vi "ev Scintilla KeyDown.vi"(4 "LF2R IDE in":refnum<class "LF2R IDE.lvclass">, 5 "Event Data":cluster{"sender":refnum<k24>, "e":refnum<k24>}, 6 "Control Ref":refnum<k24>, 7 "Event Common Data":T1) -> ()   [LabVIEW 2018, in "LF2R IDE.lvlib" / "LF2R IDE.lvclass"]
uses:
  LF2R IDE.lvclass
  D:/project/hobby/LabVIEW/LF2R/LabVIEW/Source/ScintillaNET/dll/ScintillaNET.dll
  ScintillaNET/dll/ScintillaNET.dll
  System.Windows.Forms
  C:/Program Files (x86)/National Instruments/LabVIEW 2018/vi.lib/ActorFramework/Actor/Actor.lvclass
  LF2R IDE Cmd.ctl
  <vilib>/ActorFramework/Actor/Actor.lvclass/Actor.ctl
  <vilib>/ActorFramework/Message Enqueuer/Message Enqueuer.lvclass/Message Enqueuer.ctl
  LF2R IDE Messages/LF2R IDE Cmd Msg/LF2R IDE Cmd Msg.lvclass/LF2R IDE Cmd Msg.ctl
  <vilib>/ActorFramework/Message Enqueuer/Init from Existing Queue.vi
  <vilib>/ActorFramework/Message Enqueuer/Enqueue.vi
  LF2R IDE Messages/LF2R IDE Cmd Msg/LF2R IDE Cmd Msg.lvclass
  C:/Program Files (x86)/National Instruments/LabVIEW 2018/vi.lib/ActorFramework/Message/Message.lvclass
  <vilib>/ActorFramework/Message Priority Queue/Priority Enqueue.vi
  <vilib>/ActorFramework/Message Enqueuer/Message Enqueuer.lvclass
  <vilib>/ActorFramework/Actor/Actor.lvclass
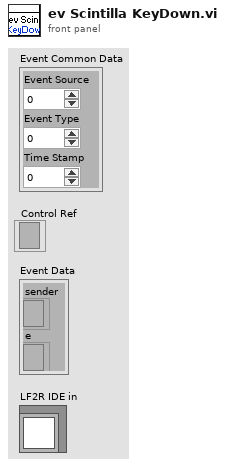
[diagram p1: front panel]
types:
  T1 = cluster{"Event Source":i32, "Event Type":u32, "Time Stamp":u32}
  T2 = typedef "LF2R IDE.lvlib/LF2R IDE.lvclass/LF2R IDE Cmd.ctl" = enum16{"Save Data File", "Write Configuration", "Save Configuration", "Update Frame Image"}
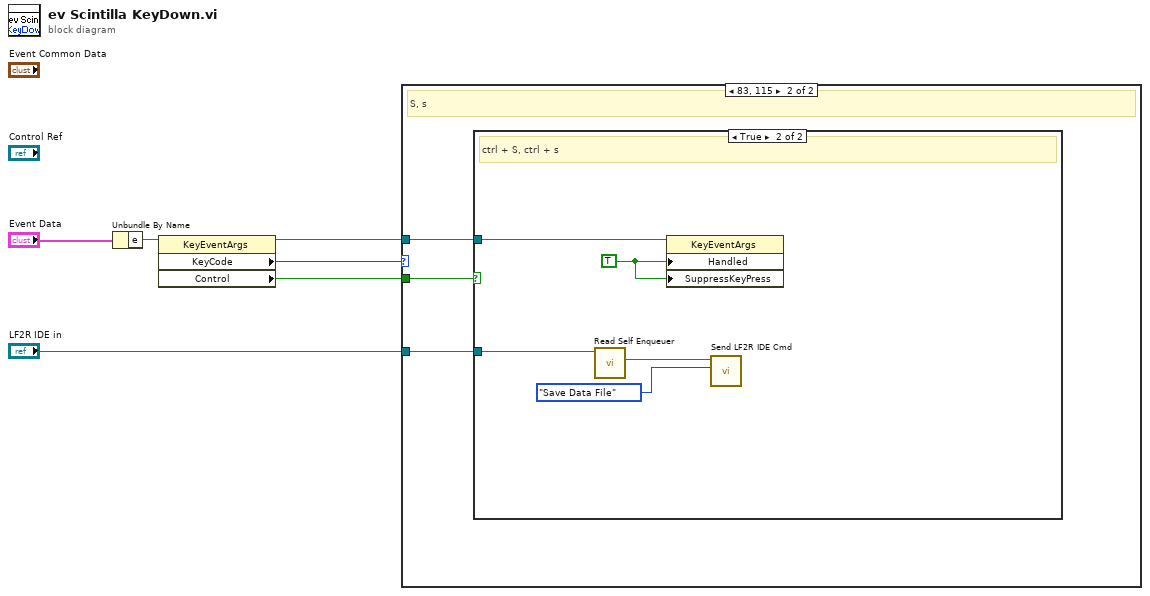
[diagram p0: block diagram]
diagram:
  n1 = Unbundle By Name("Event Data") -> ("e"=w6:refnum<k24>)
  n2 = property class="KeyEventArgs"(reference=w6) -> (reference out=w3:refnum<k24>, "KeyCode"=w5:i32, "Control"=w4:bool)  [unwired: 1 in, 1 out]
  n3 = case shown="83, 115" w5 {
    tunnel: w4 -> [_ w9]
    tunnel: w3 -> [_ w8]
    tunnel: "LF2R IDE in" -> [_ w7]
    frame 0, Default {
    }
    frame 83, 115 {
      # "S, s"
      n4 = case shown="True" w9 {
        tunnel: w8 -> [_ w14]
        tunnel: w7 -> [_ w12]
        frame False {
        }
        frame True {
          w13 = TRUE ("Handled")
          # "ctrl + S, ctrl + s"
          n5 = call <vilib>:"Read Self Enqueuer.vi"("Actor"=w12) -> ("Self Enqueuer"=w11:refnum<class "Message Enqueuer.lvclass">)  [unwired: 10 in]
          n6 = property class="KeyEventArgs"(reference=w14, "Handled"=w13, "SuppressKeyPress"=w13) -> ()  [unwired: 1 in, 2 out]
          n7 = call "Send LF2R IDE Cmd.vi"("CMD"=LF2R_IDE_Cmd."Save Data File", "Message Enqueuer"=w11) -> ()  [unwired: 8 in, 2 out]
        }
      }
    }
  }
